vi "CMD_DBSAVEASSEMBLY.vi"(6 "Gantry in":refnum<class "Gantry.lvclass">, 8 "error in (no error)":errorcluster, 10 "Arguments":string[](array[string]), 11 "gScript Interpreter in":refnum<class "gScript Interpreter.lvclass">) -> (0 "error out":errorcluster, 3 "gScript Interpreter out":refnum<class "gScript Interpreter.lvclass">, 4 "Gantry out":refnum<class "Gantry.lvclass">)   [LabVIEW 2017, in "gScript Interpreter.lvclass"]
uses:
  gScript Interpreter.lvclass
  Shared Components/Gantry Class/Gantry.lvclass
  Shared Components/External/Database/DB Component.ctl
  Shared Components/External/Database/DB Test.ctl
  Shared Components/FlexWorktable/FlexWorktable.lvclass
  Shared Components/External/Database/Database.lvlib
panel:
  in  "cancel":bool
  in  "Assembly Notes":string
  in  "Serial Number":string
  in  "Status":u16(ring) items=["assembled", "bonded", "glued"]
  in  "Assembly Summary":string
  in  "Assembly Components":T1(array[cluster])
  in  "finish":bool
  in  "Assembly Part":string(combo)
  # "(Edit only if you know what you are doing!)"
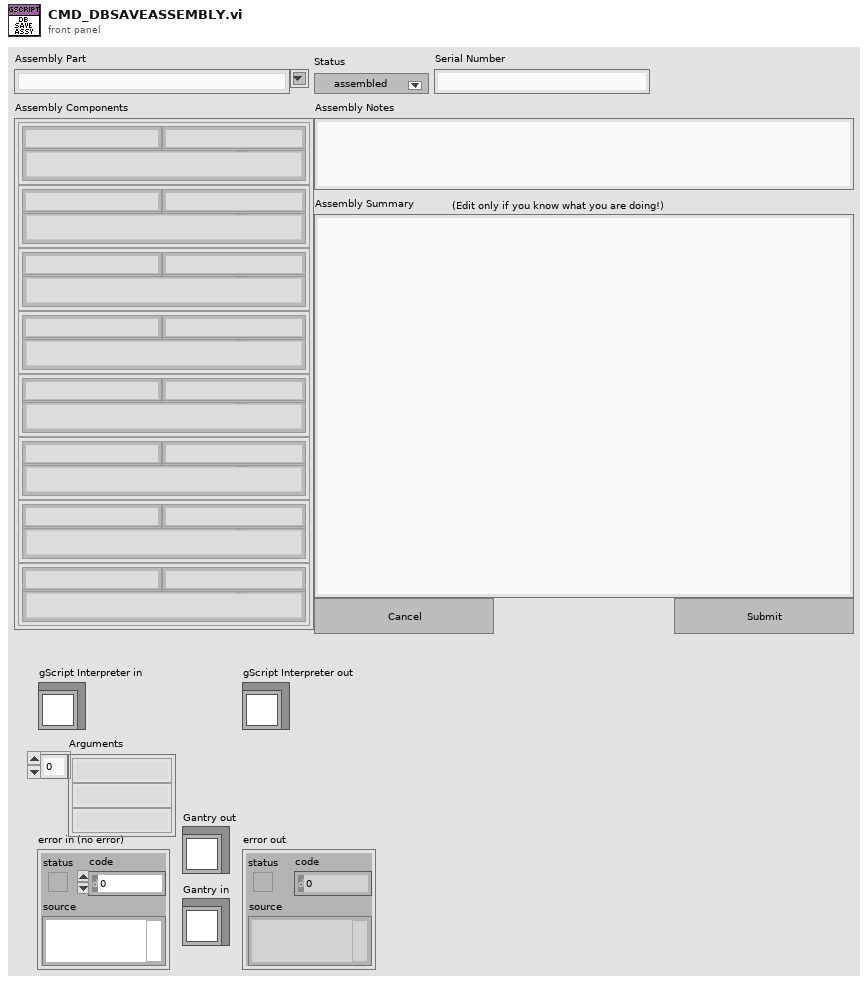
[diagram p1: front panel]
types:
  T1 = cluster{"SN":string, "Part":string, "Designation":string, "id":i32}[]
  T2 = cluster{"SN":string, "Part":string, "Designation":string, "id":i32}
  T3 = typedef "Database.lvlib/DB Test.ctl" = cluster{"description":string, "data":string, "component_id":i32, "type":string}
  T4 = typedef "Database.lvlib/DB Component.ctl" = cluster{"part":string, "version":i32, "id":i32, "status":string, "description":string, "serial_number":string, "location":string, "parent":i32}
  T5 = typedef "Database.lvlib/DB Part.ctl" = cluster{"name":string, "description":string, "version":i32, "prefix":string, "dim_x":sgl, "dim_y":sgl, "dim_z":sgl, "type":string}
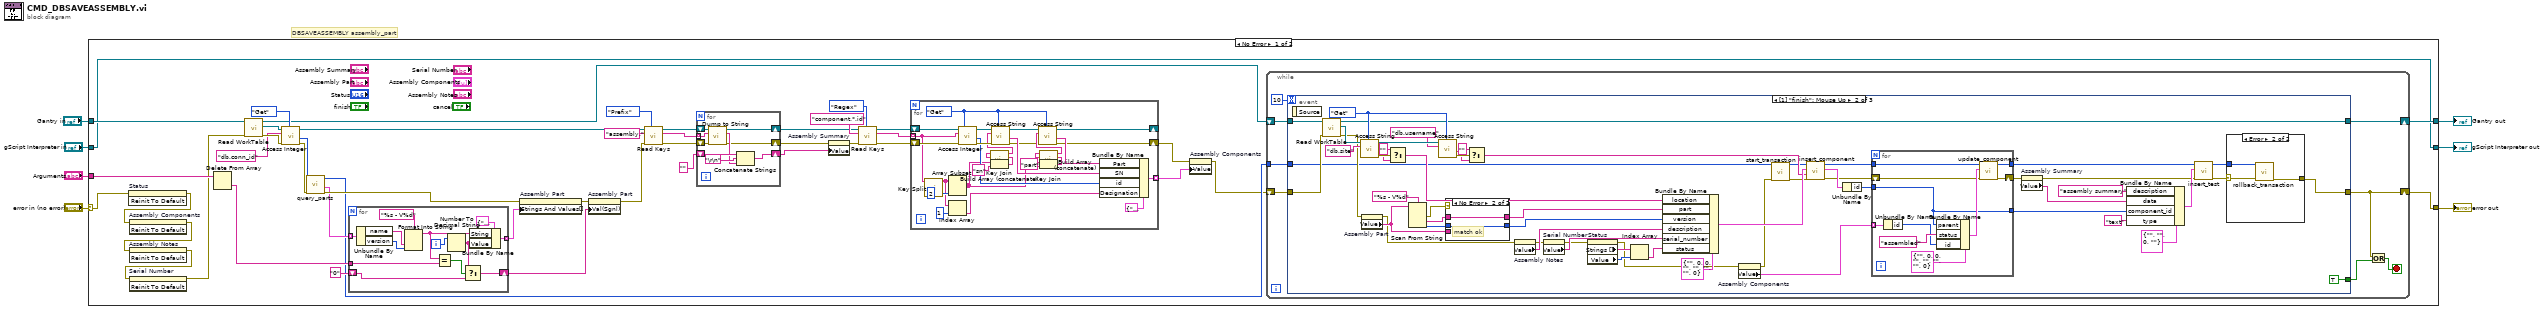
[diagram p0: block diagram]
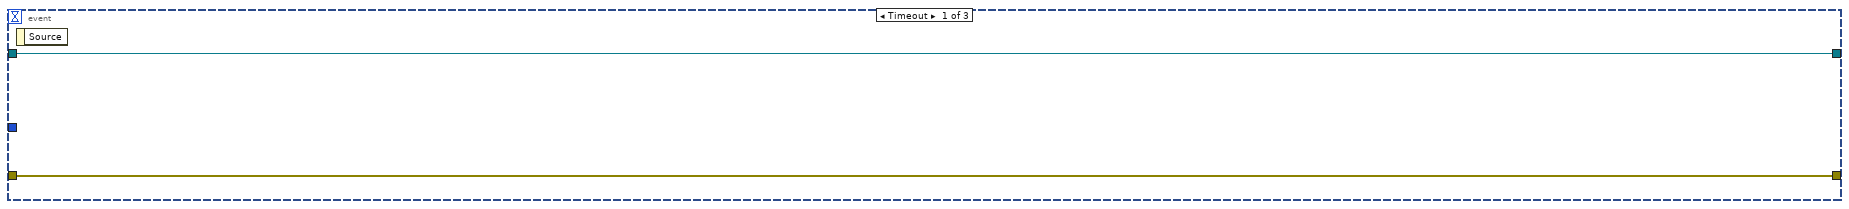
[diagram p2: hidden frame]
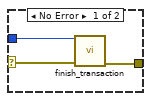
[diagram p3: hidden frame]
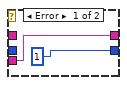
[diagram p4: hidden frame]
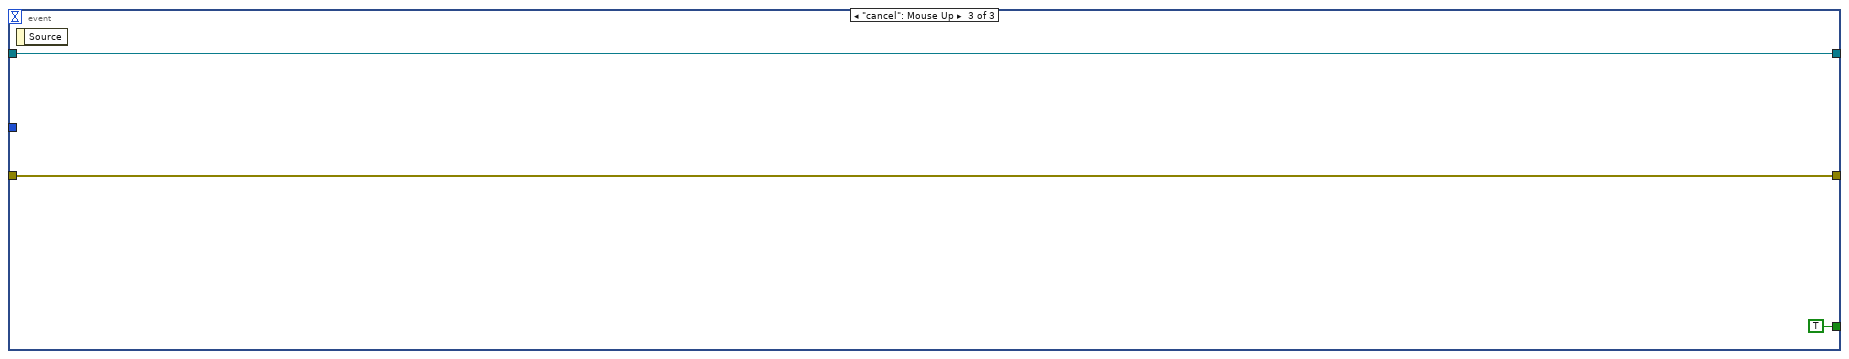
[diagram p5: hidden frame]
diagram:
  # "DBSAVEASSEMBLY assembly_part"
  n1 = case shown="No Error" "error in (no error)" {
    selector: "error in (no error)" -> [w12 w193]
    tunnel: [w39 w193] -> w6
    tunnel: [w38 w192] -> w4
    tunnel: "gScript Interpreter in" -> [w38 w192]
    tunnel: "Arguments" -> [w36 _]
    tunnel: "Gantry in" -> [w52 w191]
    tunnel: [w40 w191] -> w1
    frame No Error {
      n2 = invoke on="Status" class="Ring (strict)" method="Reinit To Default"(error in=w12) -> (error out=w11:errorcluster)  [unwired: 2 in, 2 out]
      n3 = invoke on="Assembly Components" class="Arr (strict)" method="Reinit To Default"(error in=w11) -> (error out=w10:errorcluster)  [unwired: 2 in, 2 out]
      n4 = invoke on="Assembly Notes" class="Str" method="Reinit To Default"(error in=w10) -> (error out=w9:errorcluster)  [unwired: 2 in, 2 out]
      n5 = invoke on="Serial Number" class="Str" method="Reinit To Default"(error in=w9) -> (error out=w8:errorcluster)  [unwired: 2 in, 2 out]
      n6 = Delete From Array(array=w36) -> (deleted portion=w35:string)  [unwired: 2 in, 1 out]
      n7 = call-dynamic "Read WorkTable.vi"("error in"=w8, "Gantry Class in"=w52) -> ("error out"=w49:errorcluster, "Worktable"=w51:refnum<class "FlexWorktable.lvclass">, "Gantry Class out"=w14:refnum<class "Gantry.lvclass">)  [unwired: 7 in]
      n8 = call-dynamic "Access Integer.vi"("Get/Set"=enum16{"Get", "Set"}."Get", "error in (no error)"=w49, "Key"="db.conn_id", "FlexWorktable in"=w51) -> ("error out"=w46:errorcluster, "Value out"=w47:i32, "FlexWorktable out"=w34:refnum<class "FlexWorktable.lvclass">)  [unwired: 5 in]
      n9 = call "query_parts.vi"("error in (no error)"=w46, "DB Session ID"=w47) -> ("error out"=w44:errorcluster, "Parts"=w37:T5[], "DB Session ID out"=w16:i32)  [unwired: 7 in]
      n10 = for {
        tunnel: w37 -> [w190] mode=indexing
        tunnel: [w184] -> w45 mode=indexing
        tunnel: w35 -> [w182]
        shift-right: [w179] -> w42
        shift-left: "0" -> [w180]
        i -> [w185]
        n11 = Unbundle By Name(w190) -> ("name"=w188:string, "version"=w187:i32)
        n12 = Format Into String(format string="%s - V%d", w188, w187) -> (resulting string=w183:string)  [unwired: 2 in, 1 out]
        n13 = Equal?(x=w183, y=w182) -> (x = y?=w181:bool)
        n14 = Number To Decimal String(number=w185) -> (decimal integer string=w178:string)  [unwired: 1 in]
        n15 = Select(t=w178, s=w181, f=w180) -> (s? t:f=w179:string)
        n16 = Bundle By Name(cluster=cluster{"String":string, "Value":string} {"String"="", "Value"=""}, "String"=w183, "Value"=w178) -> (w184:cluster{"String":string, "Value":string})
      }
      n17 = property on="Assembly Part" class="CmbBox"(error in=w44, "Strings And Values[]"=w45) -> (error out=w41:errorcluster)  [unwired: 1 in, 1 out]
      n18 = property on="Assembly Part" class="CmbBox"(error in=w41, "Val(Sgnl)"=w42) -> (error out=w32:errorcluster)  [unwired: 1 in, 1 out]
      n19 = call-dynamic "Read Keys.vi"("Prefix/Regex"=enum16{"Prefix", "Regex"}."Prefix", "error in (no error)"=w32, "Selector"="assembly.", "FlexWorktable in"=w34) -> ("error out"=w28:errorcluster, "Keys"=w29:string[], "FlexWorktable out"=w33:refnum<class "FlexWorktable.lvclass">)  [unwired: 5 in]
      n20 = for {
        tunnel: w29 -> [w86] mode=indexing
        shift-right: [w83] -> w25
        shift-left: "" -> [w82]
        shift-right: [w80] -> w26
        shift-left: w28 -> [w85]
        shift-right: [w79] -> w18
        shift-left: w33 -> [w87]
        n21 = call-dynamic "Dump to String.vi"("error in (no error)"=w85, "Key"=w86, "FlexWorktable in"=w87) -> ("error out"=w80:errorcluster, "Line out"=w81:string, "FlexWorktable out"=w79:refnum<class "FlexWorktable.lvclass">)  [unwired: 6 in]
        n22 = Concatenate Strings(w82, "\r\n", w81) -> (w83:string)
      }
      n23 = property on="Assembly Summary" class="Str"(error in=w26, "Value"=w25) -> (error out=w17:errorcluster)  [unwired: 1 in, 1 out]
      n24 = call-dynamic "Read Keys.vi"("Prefix/Regex"=enum16{"Prefix", "Regex"}."Regex", "error in (no error)"=w17, "Selector"="component.*.id", "FlexWorktable in"=w18) -> ("error out"=w20:errorcluster, "Keys"=w21:string[], "FlexWorktable out"=w24:refnum<class "FlexWorktable.lvclass">)  [unwired: 5 in]
      n25 = for {
        tunnel: w21 -> [w74] mode=indexing
        shift-right: [w57] -> w19
        shift-left: w20 -> [w75]
        shift-right: [w56] -> _
        shift-left: w24 -> [w76]
        tunnel: [w77] -> w15 mode=indexing
        w68 = enum16{"Get", "Set"}."Get" ("Get/Set")
        n26 = call "Key Split.vi"("Key"=w74) -> ("Key Elements"=w72:string[])  [unwired: 10 in]
        n27 = Array Subset(array=w72, length=2) -> (w53:string[])  [unwired: 1 in]
        n28 = Index Array(array=w72, index=1) -> (element=w55:string)
        n29 = call-dynamic "Access Integer.vi"("Get/Set"=w68, "error in (no error)"=w75, "Key"=w74, "FlexWorktable in"=w76) -> ("error out"=w66:errorcluster, "Value out"=w54:i32, "FlexWorktable out"=w70:refnum<class "FlexWorktable.lvclass">)  [unwired: 5 in]
        n30 = Build Array (concatenate)(w53, "sn") -> (w65:string[])
        n31 = call "Key Join.vi"("Key Elements"=w65) -> ("Key"=w64:string)  [unwired: 10 in]
        n32 = call-dynamic "Access String.vi"("Get/Set"=w68, "error in (no error)"=w66, "Key"=w64, "FlexWorktable in"=w70) -> ("error out"=w58:errorcluster, "Value out"=w60:string, "FlexWorktable out"=w69:refnum<class "FlexWorktable.lvclass">)  [unwired: 5 in]
        n33 = Build Array (concatenate)(w53, "part") -> (w62:string[])
        n34 = call "Key Join.vi"("Key Elements"=w62) -> ("Key"=w61:string)  [unwired: 10 in]
        n35 = call-dynamic "Access String.vi"("Get/Set"=w68, "error in (no error)"=w58, "Key"=w61, "FlexWorktable in"=w69) -> ("error out"=w57:errorcluster, "Value out"=w59:string, "FlexWorktable out"=w56:refnum<class "FlexWorktable.lvclass">)  [unwired: 5 in]
        n36 = Bundle By Name(cluster=T2 {"SN"="", "Part"="", "Designation"="", "id"=0} ("Selected Component"), "Part"=w59, "SN"=w60, "id"=w54, "Designation"=w55) -> (w77:T2)
      }
      n37 = property on="Assembly Components" class="Arr (strict)"(error in=w19, "Value"=w15) -> (error out=w13:errorcluster)  [unwired: 1 in, 1 out]
      n38 = while {
        shift-right: [w94] -> w40
        shift-left: w14 -> [w95]
        shift-right: [w90] -> w39
        shift-left: w13 -> [w92]
        tunnel: w16 -> [w93]
        stop <- w88 stop-if-true
        n39 = event shown="[1] \"finish\": Mouse Up" {
          selector: _ -> [_ _ _]
          dyn-events: _ -> [_ _ _]
          timeout: 10 -> [_ _ _]
          tunnel: w95 -> [w97 w153 w176]
          tunnel: [w97 w119 w176] -> w94
          tunnel: w93 -> [_ w113 _]
          tunnel: w92 -> [w96 w152 w177]
          tunnel: [w96 w99 w177] -> w90
          tunnel: [_ TRUE TRUE] -> w89
          event Timeout {
            n40 = event-data() -> ()  [unwired: 1 in, 1 out]
          }
          event "finish": Mouse Up {
            w126 = enum16{"Get", "Set"}."Get" ("Get/Set")
            n41 = event-data() -> ()  [unwired: 1 in, 1 out]
            n42 = call-dynamic "Read WorkTable.vi"("error in"=w152, "Gantry Class in"=w153) -> ("error out"=w143:errorcluster, "Worktable"=w150:refnum<class "FlexWorktable.lvclass">, "Gantry Class out"=w119:refnum<class "Gantry.lvclass">)  [unwired: 7 in]
            n43 = call-dynamic "Access String.vi"("Get/Set"=w126, "Key"="db.site", "FlexWorktable in"=w150) -> ("error out"=w148:errorcluster, "Value out"=w147:string, "FlexWorktable out"=w127:refnum<class "FlexWorktable.lvclass">)  [unwired: 6 in]
            n44 = property on="Assembly Part" class="CmbBox"(error in=w143) -> (error out=w118:errorcluster, "Value"=w140:string)  [unwired: 1 in, 1 out]
            n45 = Select(t="", s=w148, f=w147) -> (s? t:f=w145:string)
            n46 = Scan From String(format string="%s - V%d", input string=w140) -> (error out=w117:errorcluster, output 1=w142:string, output 2=w141:i32)  [unwired: 4 in, 2 out]
            n47 = call-dynamic "Access String.vi"("Get/Set"=w126, "Key"="db.username", "FlexWorktable in"=w127) -> ("error out"=w129:errorcluster, "Value out"=w124:string)  [unwired: 6 in, 1 out]
            n48 = case shown="No Error" w117 {
              tunnel: w142 -> [_ w174]
              tunnel: w141 -> [_ w173]
              tunnel: w140 -> [w172 _]
              tunnel: [w172 w174] -> w139
              tunnel: [1 w173] -> w138
              frame Error {
              }
              frame No Error {
                # "match ok"
              }
            }
            n49 = Select(t="", s=w129, f=w124) -> (s? t:f=w115:string)
            n50 = property on="Assembly Notes" class="Str"(error in=w118) -> (error out=w136:errorcluster, "Value"=w137:string)  [unwired: 1 in, 1 out]
            n51 = property on="Serial Number" class="Str"(error in=w136) -> (error out=w134:errorcluster, "Value"=w135:string)  [unwired: 1 in, 1 out]
            n52 = property on="Status" class="Ring (strict)"(error in=w134) -> (error out=w116:errorcluster, "Strings []"=w133:string[], "Value"=w132:u16)  [unwired: 1 in, 1 out]
            n53 = Index Array(array=w133, index=w132) -> (element=w131:string)
            n54 = Bundle By Name(cluster=T4 {"part"="", "version"=0, "id"=0, "status"="", "description"="", "serial_number"="", "location"="", "parent"=0} ("Component"), "location"=w145, "part"=w139, "version"=w138, "description"=w137, "serial_number"=w135, "status"=w131) -> (w130:T4)
            n55 = property on="Assembly Components" class="Arr (strict)"(error in=w116) -> (error out=w114:errorcluster, "Value"=w123:T1)  [unwired: 1 in, 1 out]
            n56 = call "start_transaction.vi"("DB Session ID"=w113, "error in (no error)"=w114) -> ("DB Session ID out"=w112:i32, "error out"=w111:errorcluster)  [unwired: 12 in]
            n57 = call "insert_component.vi"("error in (no error)"=w111, "who"=w115, "Component"=w130, "DB Session ID"=w112) -> ("error out"=w110:errorcluster, "Component out"=w121:T4, "DB Session ID out"=w122:i32)  [unwired: 5 in]
            n58 = Unbundle By Name(w121) -> ("id"=w120:i32)
            n59 = for {
              tunnel: w123 -> [w168] mode=indexing
              shift-right: [w162] -> w102
              shift-left: w110 -> [w164]
              tunnel: w122 -> [w170]
              tunnel: w120 -> [w161]
              tunnel: [w163] -> w109
              tunnel: [w161] -> w103
              n60 = Unbundle By Name(w168) -> ("id"=w166:i32)
              n61 = Bundle By Name(cluster=T4 {"part"="", "version"=0, "id"=0, "status"="", "description"="", "serial_number"="", "location"="", "parent"=0} ("Component"), "parent"=w161, "status"="assembled", "id"=w166) -> (w165:T4)
              n62 = call "update_component.vi"("error in (no error)"=w164, "Component"=w165, "DB Session ID"=w170) -> ("error out"=w162:errorcluster, "DB Session ID out"=w163:i32)  [unwired: 6 in, 1 out]
            }
            n63 = property on="Assembly Summary" class="Str"(error in=w102) -> (error out=w100:errorcluster, "Value"=w101:string)  [unwired: 1 in, 1 out]
            n64 = Bundle By Name(cluster=T3 {"description"="", "data"="", "component_id"=0, "type"=""} ("Test"), "description"="assembly summary", "data"=w101, "component_id"=w103, "type"="text") -> (w107:T3)
            n65 = call "insert_test.vi"("error in (no error)"=w100, "Test"=w107, "DB Session ID"=w109) -> ("error out"=w98:errorcluster, "DB Session ID out"=w106:i32)  [unwired: 7 in]
            n66 = case shown="Error" w98 {
              selector: w98 -> [w155 w159]
              tunnel: w106 -> [w157 w160]
              tunnel: [w156 w158] -> w99
              frame No Error {
                n67 = call "finish_transaction.vi"("DB Session ID"=w157, "error in (no error)"=w155) -> ("error out"=w156:errorcluster)  [unwired: 12 in, 1 out]
              }
              frame Error {
                n68 = call "rollback_transaction.vi"("DB Session ID"=w160, "error in (no error)"=w159) -> ("error out"=w158:errorcluster)  [unwired: 12 in, 1 out]
              }
            }
          }
          event "cancel": Mouse Up {
            n69 = event-data() -> ()  [unwired: 1 in, 1 out]
          }
        }
        n70 = Or(x=w90, y=w89) -> (x .or. y?=w88:bool)
      }
    }
    frame Error {
    }
  }
  "error out" <- w6
  "gScript Interpreter out" <- w4
  "Gantry out" <- w1
